vi "FormatString.vi"(0 "String":string, 1 "string encoding":enum16{"None", "Base64"}(ring)=enum."Base64") -> (2 "value":string)   [LabVIEW 2014, in "PythonConfiguration.lvclass"]
uses:
  PythonConfiguration.lvclass
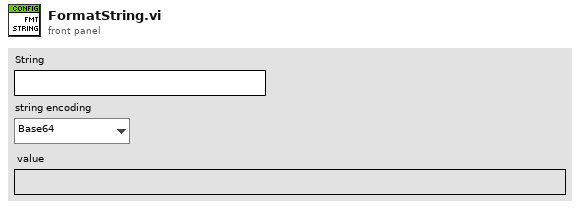
[diagram p1: front panel]
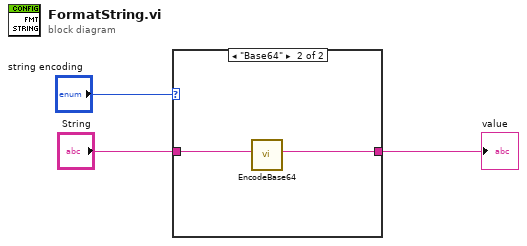
[diagram p0: block diagram]
diagram:
  n1 = case shown="\"Base64\"" "string encoding" {
    tunnel: "String" -> [w4 w6]
    tunnel: [w4 w5] -> w1
    frame "None" {
    }
    frame "Base64" {
      n2 = call "EncodeBase64.vi"("string"=w6) -> ("base64 string"=w5:string)  [unwired: 10 in]
    }
  }
  "value" <- w1
